vi "ChooseUUT.vi"(8 "error in (no error)":errorcluster, 9 "Enable":bool=TRUE, 10 "Message":string="Please select the Unit Under Test.") -> (0 "error out":errorcluster, 2 "EBAY":bool)   [LabVIEW 2017]
doc: "Displays a standard dialog box that contains an alert or a message for users.\n--------------------\n\nThis Express VI is configured as follows:\n\nMessage: Please select the Unit Under Test."
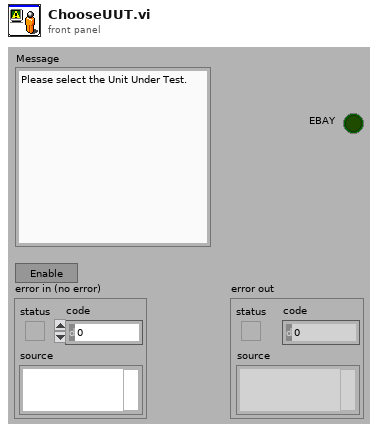
[diagram p1: front panel]
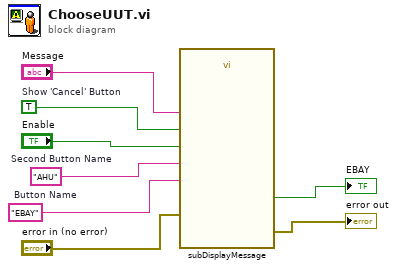
[diagram p0: block diagram]
diagram:
  w3 = "EBAY"  # Button Name
  w4 = "AHU"  # Second Button Name
  w6 = TRUE  # Show 'Cancel' Button
  n1 = call <vilib>:"subDisplayMessage.vi"("Second Button Name"=w4, "Button Name"=w3, "error in (no error)"="error in (no error)", "Enable Message"="Enable", "Show 'Cancel' Button"=w6, "Message to Display"="Message") -> ("error out"=→"error out":errorcluster, "OK?"=→"EBAY":bool)  [unwired: 4 in]
